vi "Round_to_10ns.vi"(11 "time_us":dbl) -> (3 "rounded_us":dbl)   [LabVIEW 2014]
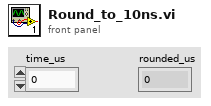
[diagram p1: front panel]
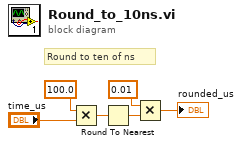
[diagram p0: block diagram]
diagram:
  # "Round to ten of ns"
  n1 = Multiply(x=100.0, y="time_us") -> (x*y=w2:dbl)
  n2 = Round To Nearest(number=w2) -> (nearest integer value=w3:dbl)
  n3 = Multiply(x=0.01, y=w3) -> (x*y=→"rounded_us":dbl)
